vi "OPC UA Server - Multiple Tags Example2.vi"() -> ()   [LabVIEW 2017]
uses:
  <vilib>/OPCUA/NI OPC UA Server.lvlib
panel:
  out "Array of NodeIds":string[](array[string])=["ns=2;s=Process Data.Temperature1", "ns=2;s=Process Data.Temperature2"]
  in  "Folder Name":string="Process Data"
  in  "Items":T1(array[cluster])=[{"name"="Temperature1", "data type"=11, "access level"=3, "description"="Simulated Temperature Values from Temperature Sensor 1"}, {"name"="Temperature2", "data type"=11, "access level"=3, "description"="Simulated Temperature Values from Temperature Sensor 2"}] {"data type" items=["Boolean"=1, "SByte"=2, "Byte"=3, "Int16"=4, "UInt16"=5, "Int32"=6, "UInt32"=7, "Int64"=8, "UInt64"=9, "Float"=10, "Double"=11, "String"=12, "DateTime"=13, "ByteString"=15, "Array of Boolean"=101, "Array of SByte"=102, "Array of Byte"=103, "Array of Int16"=104, "Array of UInt16"=105, "Array of Int32"=106, "Array of UInt32"=107, "Array of Int64"=108, "Array of UInt64"=109, "Array of Float"=110, "Array of Double"=111, "Array of String"=112, "Array of DateTime"=113, "Array of ByteString"=115]; "access level" items=["read-only"=1, "write-only"=2, "read/write"=3]}
  in  "Stop Button":bool
  out "Server Endpoint URL":string="opc.tcp://XPS15HPH:49580"
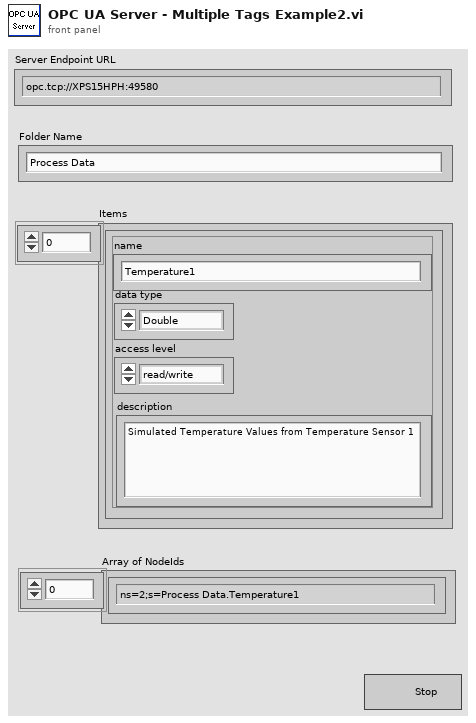
[diagram p1: front panel]
types:
  T1 = cluster{"name":string, "data type":u16, "access level":u16, "description":string}[]
  T2 = typedef "OPC UA Server Refnum.ctl" = refnum<k21>
  T3 = typedef "NodeId.ctl" = string
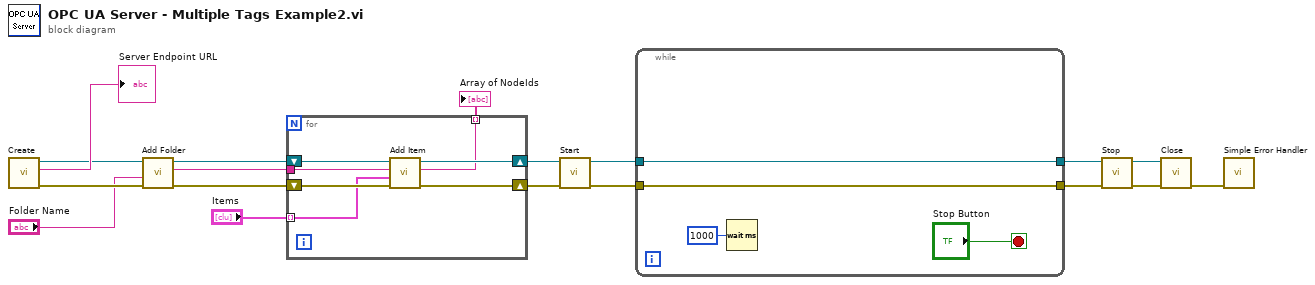
[diagram p0: block diagram]
diagram:
  n1 = call <vilib>:"Create.vi"() -> ("error out"=w18:errorcluster, "server endpoint URL"=→"Server Endpoint URL":string, "OPC UA server refnum out"=w12:T2)  [unwired: 9 in]
  n2 = call <vilib>:"Add Folder.vi"("error in (no error)"=w18, "folder name"="Folder Name", "OPC UA server refnum in"=w12) -> ("error out"=w17:errorcluster, "folder node ID"=w6:T3, "OPC UA server refnum out"=w11:T2)  [unwired: 5 in]
  n3 = for {
    tunnel: w6 -> [w23]
    shift-right: [w21] -> w4
    shift-left: w17 -> [w25]
    shift-right: [w22] -> w5
    shift-left: w11 -> [w24]
    tunnel: "Items" -> [w20] mode=indexing
    tunnel: [w19] -> w1 mode=indexing
    n4 = call <vilib>:"Add Item.vi"("error in (no error)"=w25, "item"=w20, "parent folder node ID"=w23, "OPC UA server refnum in"=w24) -> ("error out"=w21:errorcluster, "item node ID"=w19:T3, "OPC UA server refnum out"=w22:T2)  [unwired: 3 in, 1 out]
  }
  "Array of NodeIds" <- w1
  n5 = call <vilib>:"Start.vi"("error in (no error)"=w4, "OPC UA server refnum in"=w5) -> ("error out"=w16:errorcluster, "OPC UA server refnum out"=w10:T2)  [unwired: 7 in, 1 out]
  n6 = while {
    tunnel: w16 -> [w26]
    tunnel: w10 -> [w27]
    tunnel: [w27] -> w8
    tunnel: [w26] -> w7
    stop <- "Stop Button" stop-if-true
    n7 = Wait (ms)(milliseconds to wait=u32 1000) -> ()  [unwired: 1 out]
  }
  n8 = call <vilib>:"Stop.vi"("error in (no error)"=w7, "OPC UA server refnum in"=w8) -> ("error out"=w14:errorcluster, "OPC UA server refnum out"=w9:T2)  [unwired: 8 in]
  n9 = call <vilib>:"Close.vi"("error in (no error)"=w14, "OPC UA server refnum in"=w9) -> ("error out"=w13:errorcluster)  [unwired: 9 in]
  n10 = call <vilib>:"Simple Error Handler.vi"("error in (no error)"=w13) -> ()  [unwired: 4 in, 5 out]
